vi "gfitsio-not-a-refnum.vi"() -> (0 "invalid gfits refnum":T1)   [LabVIEW 2024, in "gfitsio.lvlib"]
uses:
  gfitsio.lvlib
  gfitsio-refnum.ctl
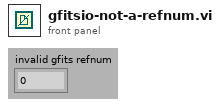
[diagram p1: front panel]
types:
  T1 = typedef "gfitsio.lvlib/gfitsio-refnum.ctl" = u64
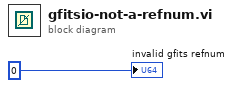
[diagram p0: block diagram]
diagram:
  "invalid gfits refnum" <- T1 0 ("GFITSIO File Refnum")
